vi "Launcher.vi"   [LabVIEW 2020, in "Application.lvclass"]
uses:
  Application.lvclass
  Container/View/View.lvclass
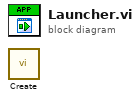
[diagram p0: block diagram]
diagram:
  n1 = call "Create.vi"() -> ()  [unwired: 10 in, 2 out]
